vi "test2.vi"() -> ()   [LabVIEW 2020]
uses:
  <vilib>/DAQmx/read.llb/DAQmx Read (Analog Wfm 1Chan NSamp).vi
  <vilib>/DAQmx/create/channels.llb/DAQmx Create Channel (AI-Voltage-Basic).vi
  <vilib>/DAQmx/configure/timing.llb/DAQmx Timing (Sample Clock).vi
  <vilib>/DAQmx/miscellaneous.llb/DAQmx Fill In Error Info.vi
panel:
  out "Waveform Chart":waveform(dbl)(graph)
  out "Time":dbl
  in  "Boolean 2":bool
  in  "Numeric":dbl
  in  "stop":bool
  out "Freq":dbl
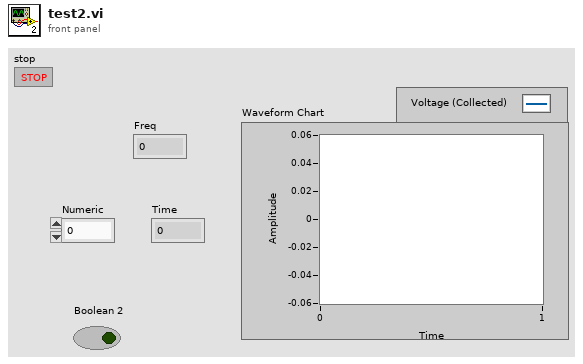
[diagram p1: front panel]
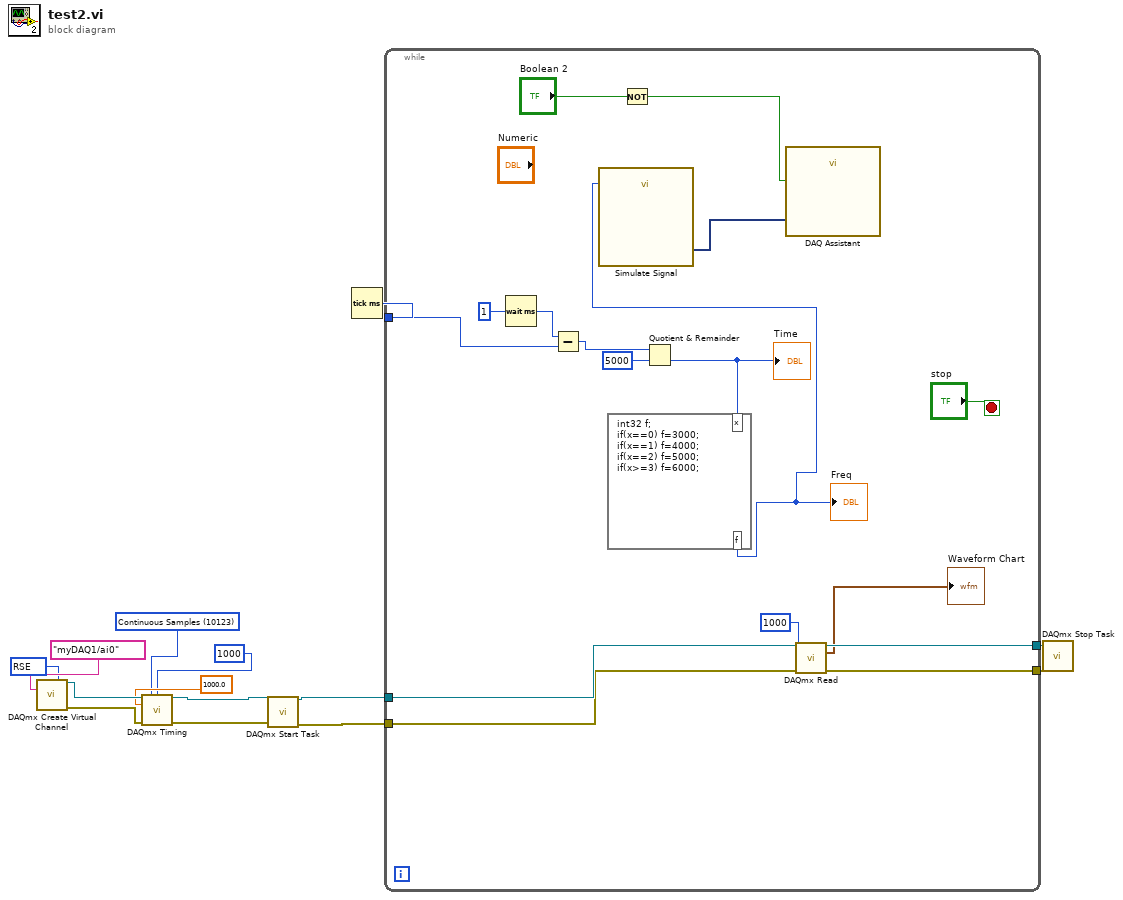
[diagram p0: block diagram]
diagram:
  w8 = 10123 items=["Finite Samples"=10178, "Continuous Samples"=10123, "Hardware Timed Single Point"=12522] ("sample mode")
  w12 = 10083 items=["Default"=-1, "RSE"=10083, "NRSE"=10078, "Differential"=10106, "Pseudodifferential"=12529] ("input terminal configuration")
  n1 = call-poly <vilib>:"DAQmx Create Virtual Channel.vi"("input terminal configuration"=w12, "physical channels"=tag "myDAQ1/ai0") -> ("task out"=w11:refnum<k21>, "error out"=w10:errorcluster)  [unwired: 12 in]
  n2 = call-poly <vilib>:"DAQmx Timing.vi"("task/channels in"=w11, "sample mode"=w8, "samples per channel"=1000, "rate"=1000.0, "error in"=w10) -> ("task out"=w6:refnum<k21>, "error out"=w5:errorcluster)  [unwired: 9 in]
  n3 = call <vilib>:"DAQmx Start Task.vi"("task/channels in"=w6, "error in"=w5) -> ("task out"=w4:refnum<k21>, "error out"=w3:errorcluster)  [unwired: 12 in]
  n4 = Tick Count (ms)() -> (millisecond timer value=w14:u32)
  n5 = while {
    tunnel: w14 -> [w25]
    tunnel: w4 -> [w19]
    tunnel: w3 -> [w18]
    tunnel: [w17] -> w2
    tunnel: [w16] -> w1
    stop <- "stop" stop-if-true
    n6 = Wait (ms)(milliseconds to wait=u32 1) -> (millisecond timer value=w26:u32)
    n7 = Subtract(x=w26, y=w25) -> (x-y=w24:u32)
    n8 = Not(x="Boolean 2") -> (.not. x?=w30:bool)
    n9 = Quotient & Remainder(x=w24, y=u32 5000) -> (floor(x/y)=w22:u32)  [unwired: 1 out]
    "Time" <- w22
    n10 = formula code="int32 f;\nif(x==0) f=3000;\nif(x==1) f=4000;\nif(x==2) f=5000;\nif(x>=3) f=6000;"("x"=w22) -> ("f"=w21:i32)
    "Freq" <- w21
    n11 = call "Simulate Signal"("Frequency"=w21) -> ("Sine"=w28:dynamicdata)  [unwired: 13 in, 1 out]
    n12 = call "DAQ Assistant"("data"=w28, "stop (F)"=w30) -> ()  [unwired: 15 in, 3 out]
    n13 = call-poly <vilib>:"DAQmx Read.vi"("task/channels in"=w19, "number of samples per channel"=1000, "error in"=w18) -> ("task out"=w17:refnum<k21>, "data"=→"Waveform Chart":waveform(dbl), "error out"=w16:errorcluster)  [unwired: 10 in]
  }
  n14 = call <vilib>:"DAQmx Stop Task.vi"("task/channels in"=w2, "error in"=w1) -> ()  [unwired: 12 in, 2 out]
